vi "Day 8 Structural Pattern Exercises.vi"() -> ()   [LabVIEW 2026]
panel:
  in  "x 2":i32=2
  in  "x":i32=6
  out "Visual Display Terminal 6":string
  out "Visual Display Terminal 5":string
  out "Visual Display Terminal 4":string
  out "Visual Display Terminal 3":string
  out "Visual Display Terminal":string
  # "[M] Reproduce the letter-pyramid pattern (A B C D E F → A → A B C D E F) \nusing nested loops and string building."
  # "[E] Print a right triangle of A B C D E growing by one letter each row."
  # "[M] Reproduce the letter-pyramid pattern (A → A B C D E → A) \nusing nested loops and string building."
  # "[M] Reproduce the letter-pyramid pattern (A B C D E F → A → A → A B C D E F) \nusing nested loops and string building."
  # "[H] Make the pattern width configurable via a front-panel control (N letters)."
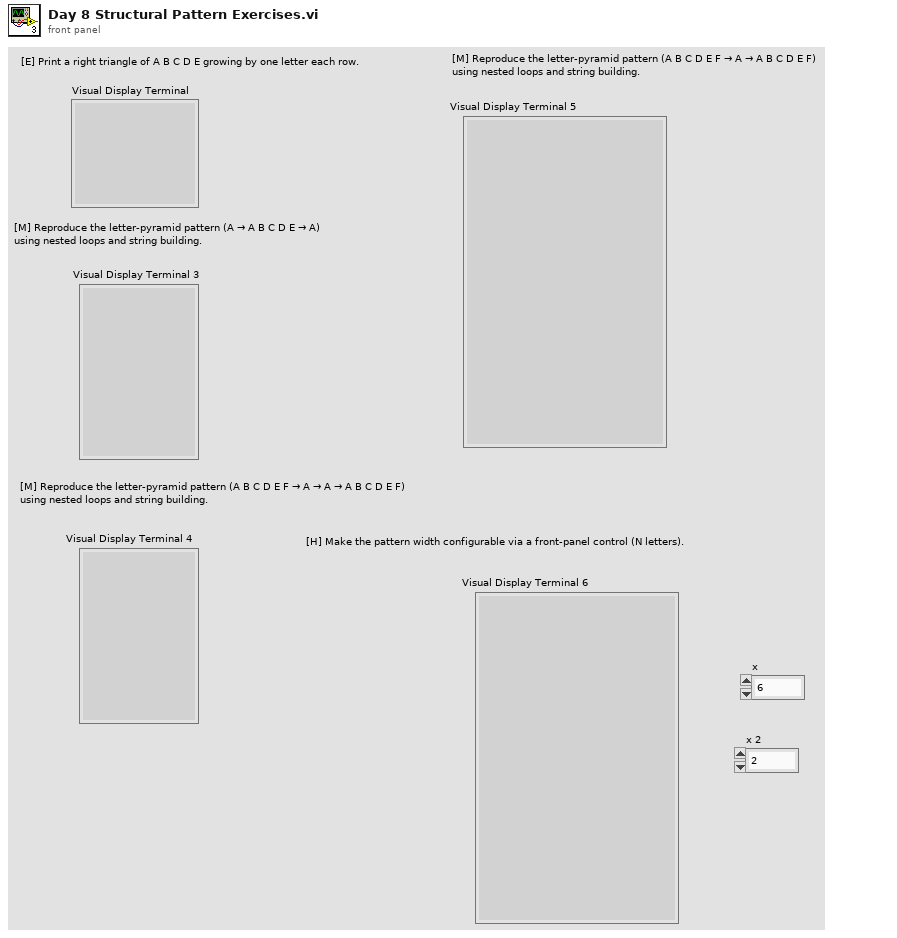
[diagram p1: front panel]
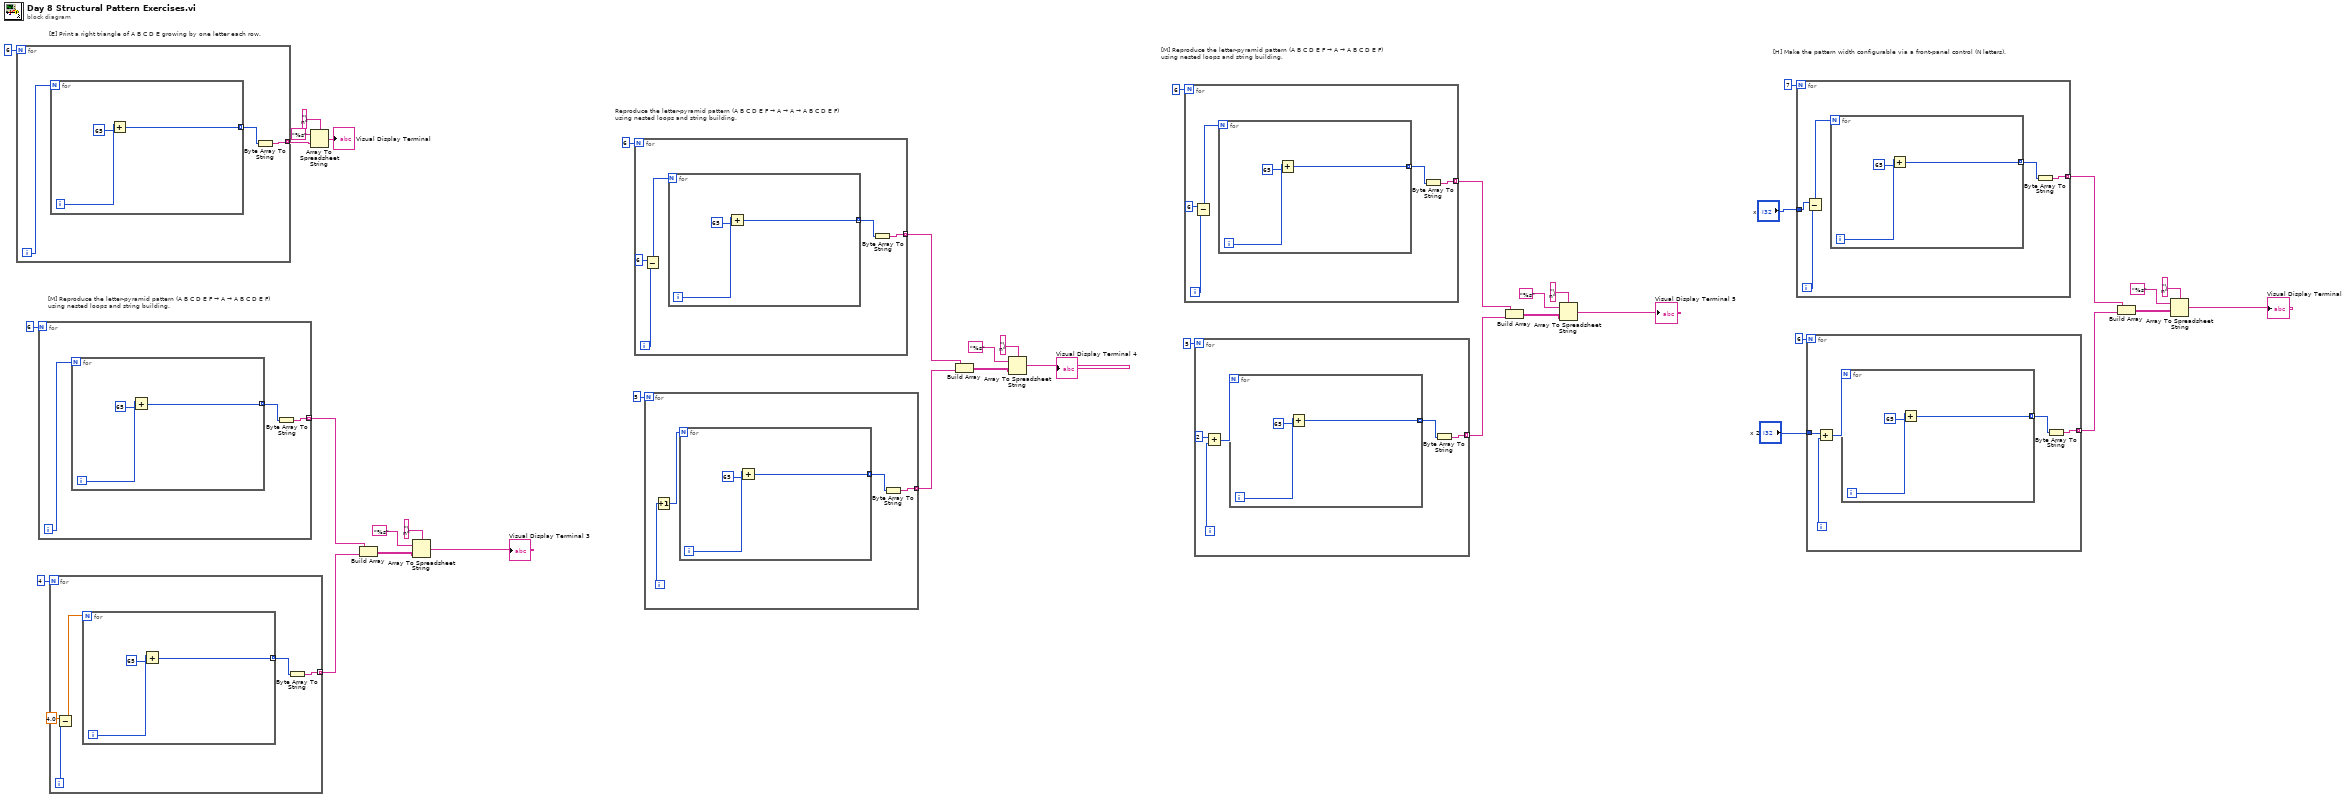
[diagram p0: block diagram]
diagram:
  # "[H] Make the pattern width configurable via a front-panel control (N letters)."
  # "[M] Reproduce the letter-pyramid pattern (A B C D E F → A → A B C D E F) \nusing nested loops and string building."
  # "Reproduce the letter-pyramid pattern (A B C D E F → A → A → A B C D E F) \nusing nested loops and string building."
  # "[M] Reproduce the letter-pyramid pattern (A B C D E F → A → A B C D E F) \nusing nested loops and string building."
  # "[E] Print a right triangle of A B C D E growing by one letter each row."
  n1 = for {
    N: 6 -> [_]
    tunnel: [w40] -> w38 mode=indexing
    i -> [w42]
    n2 = for {
      N: w42 -> [_]
      tunnel: [w43] -> w41 mode=indexing
      i -> [w45]
      n3 = Add(x=w45, y=65) -> (x+y=w43:i32)
    }
    n4 = Byte Array To String(unsigned byte array=w41) -> (string=w40:string)
  }
  n5 = for {
    N: 6 -> [_]
    tunnel: [w46] -> w30 mode=indexing
    i -> [w48]
    n6 = for {
      N: w48 -> [_]
      tunnel: [w49] -> w47 mode=indexing
      i -> [w51]
      n7 = Add(x=w51, y=65) -> (x+y=w49:i32)
    }
    n8 = Byte Array To String(unsigned byte array=w47) -> (string=w46:string)
  }
  n9 = for {
    N: 4 -> [_]
    tunnel: [w55] -> w31 mode=indexing
    i -> [w53]
    n10 = Subtract(x=4.0, y=w53) -> (x-y=w52:dbl)
    n11 = for {
      N: w52 -> [_]
      tunnel: [w57] -> w56 mode=indexing
      i -> [w59]
      n12 = Add(x=w59, y=65) -> (x+y=w57:i32)
    }
    n13 = Byte Array To String(unsigned byte array=w56) -> (string=w55:string)
  }
  n14 = Array To Spreadsheet String(delimiter (Tab)="\n", array=w38, 3:"%s" ("format string")) -> (spreadsheet string=→"Visual Display Terminal":string)
  n15 = Build Array(w30, w31) -> (w29:string[][])
  n16 = Array To Spreadsheet String(delimiter (Tab)="\n", array=w29, 3:"%s" ("format string")) -> (spreadsheet string=→"Visual Display Terminal 3":string)
  n17 = for {
    N: 6 -> [_]
    tunnel: [w63] -> w23 mode=indexing
    i -> [w62]
    n18 = Subtract(x=6, y=w62) -> (x-y=w60:i32)
    n19 = for {
      N: w60 -> [_]
      tunnel: [w65] -> w64 mode=indexing
      i -> [w67]
      n20 = Add(x=w67, y=65) -> (x+y=w65:i32)
    }
    n21 = Byte Array To String(unsigned byte array=w64) -> (string=w63:string)
  }
  n22 = for {
    N: 5 -> [_]
    tunnel: [w70] -> w11 mode=indexing
    i -> [w69]
    n23 = Increment(x=w69) -> (x+1=w68:i32)
    n24 = for {
      N: w68 -> [_]
      tunnel: [w72] -> w71 mode=indexing
      i -> [w74]
      n25 = Add(x=w74, y=65) -> (x+y=w72:i32)
    }
    n26 = Byte Array To String(unsigned byte array=w71) -> (string=w70:string)
  }
  n27 = Build Array(w23, w11) -> (w22:string[][])
  n28 = Array To Spreadsheet String(delimiter (Tab)="\n", array=w22, 3:"%s" ("format string")) -> (spreadsheet string=→"Visual Display Terminal 4":string)
  n29 = for {
    N: 6 -> [_]
    tunnel: [w78] -> w15 mode=indexing
    i -> [w77]
    n30 = Subtract(x=6, y=w77) -> (x-y=w75:i32)
    n31 = for {
      N: w75 -> [_]
      tunnel: [w80] -> w79 mode=indexing
      i -> [w82]
      n32 = Add(x=w82, y=65) -> (x+y=w80:i32)
    }
    n33 = Byte Array To String(unsigned byte array=w79) -> (string=w78:string)
  }
  n34 = for {
    N: 5 -> [_]
    tunnel: [w86] -> w16 mode=indexing
    i -> [w85]
    n35 = Add(x=2, y=w85) -> (x+y=w83:i32)
    n36 = for {
      N: w83 -> [_]
      tunnel: [w88] -> w87 mode=indexing
      i -> [w90]
      n37 = Add(x=w90, y=65) -> (x+y=w88:i32)
    }
    n38 = Byte Array To String(unsigned byte array=w87) -> (string=w86:string)
  }
  n39 = Build Array(w15, w16) -> (w14:string[][])
  n40 = Array To Spreadsheet String(delimiter (Tab)="\n", array=w14, 3:"%s" ("format string")) -> (spreadsheet string=→"Visual Display Terminal 5":string)
  n41 = for {
    N: 7 -> [_]
    tunnel: [w94] -> w6 mode=indexing
    tunnel: "x" -> [w91]
    i -> [w93]
    n42 = Subtract(x=w91, y=w93) -> (x-y=w92:i32)
    n43 = for {
      N: w92 -> [_]
      tunnel: [w96] -> w95 mode=indexing
      i -> [w98]
      n44 = Add(x=w98, y=65) -> (x+y=w96:i32)
    }
    n45 = Byte Array To String(unsigned byte array=w95) -> (string=w94:string)
  }
  n46 = for {
    N: 6 -> [_]
    tunnel: [w102] -> w7 mode=indexing
    tunnel: "x 2" -> [w99]
    i -> [w101]
    n47 = Add(x=w99, y=w101) -> (x+y=w100:i32)
    n48 = for {
      N: w100 -> [_]
      tunnel: [w104] -> w103 mode=indexing
      i -> [w106]
      n49 = Add(x=w106, y=65) -> (x+y=w104:i32)
    }
    n50 = Byte Array To String(unsigned byte array=w103) -> (string=w102:string)
  }
  n51 = Build Array(w6, w7) -> (w5:string[][])
  n52 = Array To Spreadsheet String(delimiter (Tab)="\n", array=w5, 3:"%s" ("format string")) -> (spreadsheet string=→"Visual Display Terminal 6":string)
